vi "Teleop.vi"(10 "Match Info":T1={"Autonomous Elapsed Seconds"=0.0, "TeleOp Elapsed Seconds"=0.0, "Disabled Elapsed Seconds"=0.0, "Visited Autonomous"=FALSE, "Visited TeleOp"=FALSE, "Visited Disabled"=FALSE, "Autonomous Settings"={"Autonomous Style"=enum."Independent", "VI Refnum"=refnum}}, 11 "Call Context":T2) -> ()   [LabVIEW 2014]
doc: "This VI is called for each TeleOp packet received from the DS where the robot is not disabled. It is often used to read from the joysticks and update I/O or to update setpoints for timed control loops. It should complete and return within 20 milliseconds or it may miss DS packets."
uses:
  <vilib>/Rock Robotics/WPI/DriverStation/WPI_DriverStationDerivedRobotMode.ctl
  <vilib>/Rock Robotics/WPI/DriverStation/WPI_DriverStationMatch Info.ctl
  <vilib>/Rock Robotics/WPI/Solenoid/WPI_SolenoidValue.ctl
  <vilib>/Rock Robotics/WPI/Joystick/WPI_JoystickGetSetRefNum.vi
  Robot Global Data.vi
  Gyro/Gyro Global.vi
  <vilib>/Rock Robotics/WPI/Solenoid/WPI_SolenoidSetEnum.vi
  navX-MXP Library/navX-MXP IMU.lvlib
panel:
  out "error out":errorcluster
  out "up":bool
  out "same":bool
  out "manual?":bool
  out "t?":bool
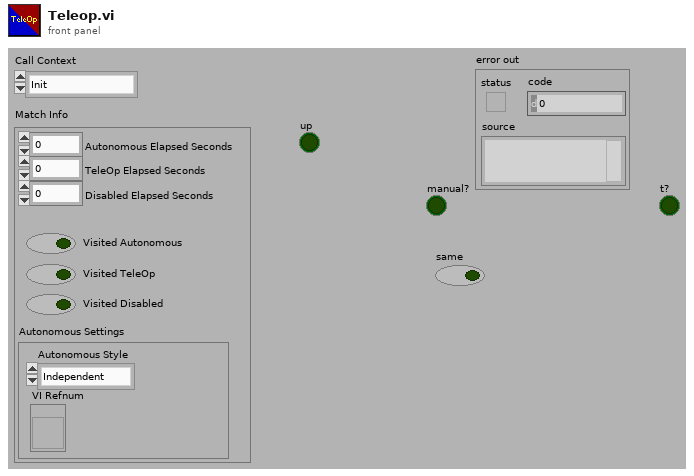
[diagram p1: front panel]
types:
  T1 = typedef "WPI_DriverStationMatch Info.ctl" = cluster{"Autonomous Elapsed Seconds":dbl, "TeleOp Elapsed Seconds":dbl, "Disabled Elapsed Seconds":dbl, "Visited Autonomous":bool, "Visited TeleOp":bool, "Visited Disabled":bool, "Autonomous Settings":cluster{"Autonomous Style":enum16{"Iterative", "Independent"}, "VI Refnum":refnum<vi>}}
  T2 = typedef "WPI_DriverStationDerivedRobotMode.ctl" = enum16{"Init", "Execute", "Stop"}
  T3 = typedef "WPI_SolenoidValue.ctl" = enum16{"Off", "On", "Forward", "Reverse"}
  T4 = typedef "WPI_JoystickDevRef.ctl" = cluster{"Device":T5}
  T5 = typedef "WPI_JoystickDeviceEnum.ctl" = enum16{"USB 0", "USB 1", "USB 2", "USB 3", "USB 4", "USB 5"}
  T6 = typedef "WPI_MotorControlDeviceRef.ctl" = cluster{"DeviceStatus":errorcluster, "Type":T7, "PWM":cluster{"Controller":T8, "PWM Channel":T9, "DeadBand":T10}, "CAN":cluster{"Device Number":u8, "Control Mode":T11, "Semaphore":T12, "Max Vout":dbl, "TalonSRX Control Mode":T13}, "Invert":bool, "TransformRef":T14, "InvTransformRef":T14}
  T7 = typedef "WPI_MotorControlType.ctl" = enum16{"PWM", "CAN", "CANTalonSRX"}
  T8 = typedef "FPGA_TypedefDigitalModule.ctl" = enum16{"Controller 1"}
  T9 = typedef "FPGA_DIOPWMChannel.ctl" = enum8{"PWM 0", "PWM 1", "PWM 2", "PWM 3", "PWM 4", "PWM 5", "PWM 6", "PWM 7", "PWM 8", "PWM 9", "PWM MXP 0", "PWM MXP 1", "PWM MXP 2", "PWM MXP 3", "PWM MXP 4", "PWM MXP 5", "PWM MXP 6", "PWM MXP 7", "PWM MXP 8", "PWM MXP 9", "Invalid"}
  T10 = typedef "WPI_PWMDeadband.ctl" = cluster{"Name":string, "maxPositivePwm":i32, "minPositivePwm":i32, "centerPwm":i32, "maxNegativePwm":i32, "minNegativePwm":i32, "angularRange":u16}
  T11 = typedef "WPI_CANJaguar_ControlMode.ctl" = enum8{"Percent VBus", "Current", "Speed", "Position", "Voltage"}
  T12 = typedef "Semaphore RefNum" = refnum<k1>
  T13 = typedef "WPI_CANTalonSRX_APIControlMode.ctl" = enum8{"Percent VBus", "Speed", "Position", "Slave", "Unchanged / Invalid"}
  T14 = typedef "WPI_PWMTransform_ConPane.ctl" = refnum<vi>
  T15 = typedef "navX-MXP IMU.lvlib/navX SPI DevRef.ctl" = cluster{"SPIDevRef":T16, "Board Information":T18, "Status":T19, "Offsets":cluster{"Yaw":dbl, "Quat W":dbl, "Quat X":dbl, "Quat Y":dbl, "Quat Z":dbl}, "Update Rate (4Hz-60Hz)":u8, "refnum name":string, "error":errorcluster}
  T16 = typedef "WPI_SPIDevRef.ctl" = cluster{"DevStatus":errorcluster, "Handle":i32, "Controller":T8, "SPI Bus":T17}
  T17 = typedef "spi_bus.ctl" = enum16{"SPI On-Board, CS0", "SPI On-Board, CS1", "SPI On-Board, CS2", "SPI On-Board, CS3", "SPI MXP", "Invalid"}
  T18 = typedef "navX-MXP IMU.lvlib/navX Board Information.ctl" = cluster{"WhoAmI (50 | 0x32)":u8, "Board Revision":u8, "Firmware Major Version":u8, "Firmware Minor Version":u8}
  T19 = typedef "navX-MXP IMU.lvlib/navX Status Data.ctl" = cluster{"Update Rate Hz":u8, "Accelerometer Full-Scale Range":u8, "Gyro Full-Scale Range":u16, "NAVX_OP_STATUS":T20, "NAVX_CAL_STATUS":T21, "NAVX_SELFTEST_STATUS":u8, "NAVX_SENSOR_STATUS":T22}
  T20 = typedef "navX-MXP IMU.lvlib/navX NAVX_OP_STATUS.ctl" = u8
  T21 = typedef "navX-MXP IMU.lvlib/navX NAVX_CAL_STATUS.ctl" = u8
  T22 = typedef "navX-MXP IMU.lvlib/navX NAVX_SENSOR_STATUS.ctl" = cluster{"MOVING":bool, "YAW_STABLE":bool, "MAG_DISTURBANCE":bool, "ALTITUDE_VALID":bool, "SEALEVEL_PRESS_SET":bool, "FUSED_HEADING_VALID":bool}
  T23 = typedef "navX-MXP IMU.lvlib/navX YPRH Data.ctl" = cluster{"Yaw":dbl, "Pitch":dbl, "Roll":dbl, "Heading":dbl}
  T24 = typedef "WPI_EncoderDevRef.ctl" = cluster{"DevStatus":errorcluster, "EncoderIndex":T25, "CounterIndex":T26, "DistancePerCount":dbl, "Decoding Type":T27}
  T25 = typedef "FPGA_EncoderIdx.ctl" = enum8{"Enc 0", "Enc 1", "Enc 2", "Enc 3", "Enc 4", "Enc 5", "Enc 6", "Enc 7", "Invalid"}
  T26 = typedef "FPGA_CounterCtrSystemIndex.ctl" = enum8{"Ctr 0", "Ctr 1", "Ctr 2", "Ctr 3", "Ctr 4", "Ctr 5", "Ctr 6", "Ctr 7", "Invalid"}
  T27 = typedef "WPI_EncoderType.ctl" = enum16{"1x", "2x", "4x"}
  T28 = typedef "WPI_SolenoidDevRef.ctl" = cluster{"DevStatus":errorcluster, "Pneumatics Control Module":u8, "Forward Solenoid Channel":T29, "Reverse Solenoid Channel":T29}
  T29 = typedef "WPI_SolenoidChannel.ctl" = enum8{"Solenoid 0", "Solenoid 1", "Solenoid 2", "Solenoid 3", "Solenoid 4", "Solenoid 5", "Solenoid 6", "Solenoid 7", "Invalid"}
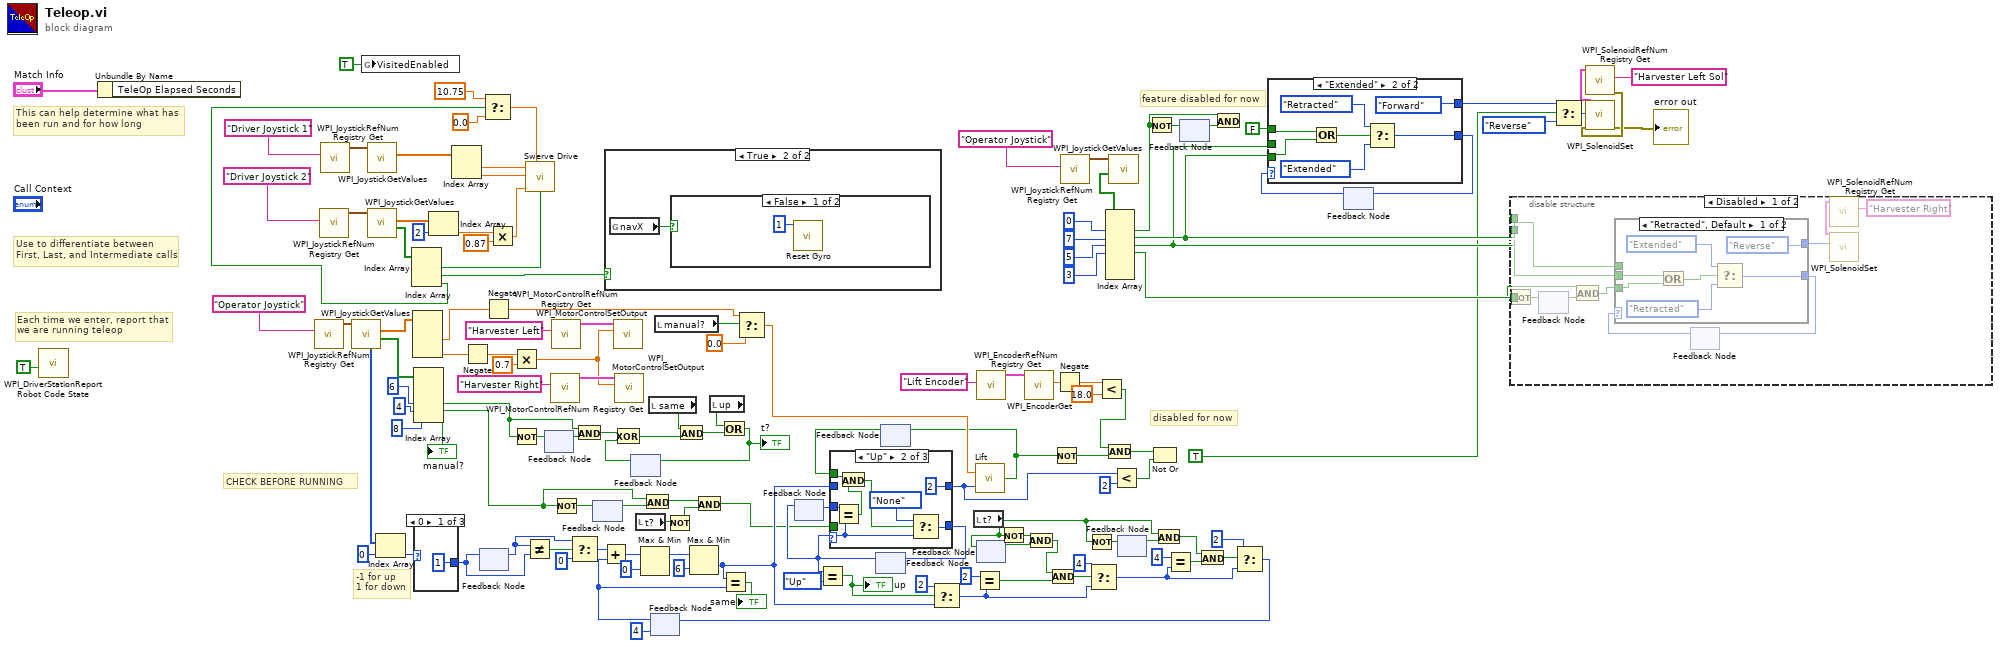
[diagram p0: block diagram]
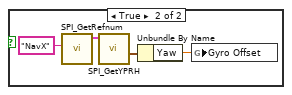
[diagram p3: hidden frame]
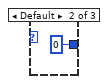
[diagram p4: hidden frame]
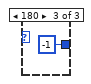
[diagram p5: hidden frame]
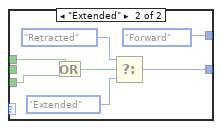
[diagram p6: hidden frame]
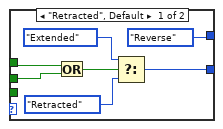
[diagram p8: hidden frame]
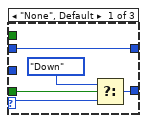
[diagram p9: hidden frame]
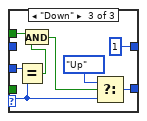
[diagram p10: hidden frame]
diagram:
  # "disabled for now"
  # "feature disabled for now"
  # "CHECK BEFORE RUNNING"
  # "-1 for up\n1 for down"
  # "Each time we enter, report that\nwe are running teleop"
  # "Use to differentiate between\nFirst, Last, and Intermediate calls"
  # "This can help determine what has\nbeen run and for how long"
  n1 = call <vilib>:"WPI_DriverStationReport Robot Code State.vi"("TeleOp"=TRUE ("Autonomous")) -> ()  [unwired: 10 in, 1 out]
  n2 = Unbundle By Name("Match Info") -> ()  [unwired: 1 out]
  n3 = call <vilib>:"WPI_JoystickRefNum Registry Get.vi"("refnum name"="Operator Joystick") -> ("JoystickDevRef"=w125:T4)  [unwired: 1 in, 9 out]
  n4 = call <vilib>:"WPI_JoystickRefNum Registry Get.vi"("refnum name"="Driver Joystick 2") -> ("JoystickDevRef"=w133:T4)  [unwired: 1 in, 9 out]
  n5 = call <vilib>:"WPI_JoystickRefNum Registry Get.vi"("refnum name"="Driver Joystick 1") -> ("JoystickDevRef"=w135:T4)  [unwired: 1 in, 9 out]
  n6 = call <vilib>:"WPI_JoystickGetValues.vi"("JoystickDevRef"=w125) -> ("Buttons"=w112:bool[], "Axes"=w124:dbl[], "POVs"=w119:i16[])  [unwired: 6 in, 2 out]
  n7 = global write "Gyro Global.vi" "VisitedEnabled"(TRUE ("VisitedEnabled")) -> ()
  n8 = call <vilib>:"WPI_JoystickGetValues.vi"("JoystickDevRef"=w135) -> ("Axes"=w131:dbl[])  [unwired: 6 in, 4 out]
  n9 = call <vilib>:"WPI_JoystickGetValues.vi"("JoystickDevRef"=w133) -> ("Buttons"=w127:bool[], "Axes"=w129:dbl[])  [unwired: 6 in, 3 out]
  n10 = Index Array(array=w119, index=0) -> (element=w44:i16)
  n11 = Index Array(array=w127) -> (element #1=w22:bool, element #2=w19:bool, element #3=w6:bool)  [unwired: 3 in]
  n12 = Index Array(array=w124) -> (element #2=w108:dbl, element #4=w109:dbl)  [unwired: 4 in, 2 out]
  n13 = Index Array(array=w112, index #3=6 ("index"), index #4=4 ("index"), index #5=8 ("index")) -> (element #3=w48:bool, element #4=w103:bool, element #5=→"manual?":bool)  [unwired: 2 in, 2 out]
  n14 = case shown="0" w44 {
    tunnel: [1 0 -1] -> w43
    frame 0 {
    }
    frame Default {
    }
    frame 180 {
    }
  }
  n15 = Index Array(array=w129, index=2) -> (element=w3:dbl)
  n16 = Index Array(array=w131) -> (element #1=w120:dbl, element #2=w130:dbl)  [unwired: 2 in]
  n17 = Negate(x=w109) -> (-x=w78:dbl)
  n18 = feedback-in #1(w43) -> ()
  n19 = feedback #1() -> (w45:i32)  [unwired: 1 in]
  n20 = Select(t=10.75 ("Rot. Point Y"), s=w6, f=0.0) -> (s? t:f=w4:dbl)
  n21 = Negate(x=w108) -> (-x=w73:dbl)
  n22 = Multiply(x=w3, y=0.87) -> (x*y=w2:dbl)
  n23 = Multiply(x=w78, y=0.7) -> (x*y=w21:dbl)
  n24 = Not(x=w48) -> (.not. x?=w82:bool)
  n25 = Not Equal?(x=w45, y=w43) -> (x != y?=w117:bool)
  n26 = call "Swerve Drive.vi"("X"=w120, "Rot. Point Y"=w4, "Y"=w130, "Z"=w2, "Robot-Centric"=w22) -> ()  [unwired: 11 in]
  n27 = feedback #2() -> (w83:bool)  [unwired: 1 in]
  n28 = feedback-in #2(w82) -> ()
  n29 = call <vilib>:"WPI_MotorControlRefNum Registry Get.vi"("refnum name"="Harvester Right") -> ("MotorControlDevRef"=w121:T6)  [unwired: 9 in, 1 out]
  n30 = call <vilib>:"WPI_MotorControlRefNum Registry Get.vi"("refnum name"="Harvester Left") -> ("MotorControlDevRef"=w122:T6)  [unwired: 9 in, 1 out]
  n31 = Not(x=w103) -> (.not. x?=w105:bool)
  n32 = Select(t=w45, s=w117, f=i16 0) -> (s? t:f=w52:i32)
  n33 = And(x=w48, y=w83) -> (x .and. y?=w81:bool)
  n34 = feedback #3() -> (w104:bool)  [unwired: 1 in]
  n35 = feedback-in #3(w105) -> ()
  n36 = case shown="True" w19 {
    frame False {
    }
    frame True {
      n37 = global read "Robot Global Data.vi" "navX"() -> (w141:bool)
      n38 = case shown="False" w141 {
        frame False {
          n39 = call "Reset Gyro.vi"("Gyro ID (1 or 2)"=1) -> ()  [unwired: 11 in]
        }
        frame True {
          n40 = call "SPI_GetRefnum.vi"("refnum name"="NavX") -> ("navX DevRef"=w144:T15)  [unwired: 9 in, 1 out]
          n41 = call "SPI_GetYPRH.vi"("navX DevRef"=w144) -> ("YPRH"=w143:T23)  [unwired: 8 in, 2 out]
          n42 = Unbundle By Name(w143) -> ("Yaw"=w146:dbl)
          n43 = global write "Robot Global Data.vi" "Gyro Offset"(w146) -> ()
        }
      }
    }
  }
  n44 = call <vilib>:"WPI_MotorControlSetOutput.vi"("Output"=w21, "MotorControlDevRef"=w122) -> ()  [unwired: 7 in, 3 out]
  n45 = call <vilib>:"WPI_MotorControlSetOutput.vi"("Output"=w21, "MotorControlDevRef"=w121) -> ()  [unwired: 7 in, 3 out]
  n46 = feedback #4() -> (w80:bool)  [unwired: 1 in]
  n47 = Exclusive Or(1:w80, 2:w81) -> (0:w36:bool)
  n48 = local read "t?"() -> (w28:bool)
  n49 = And(x=w103, y=w104) -> (x .and. y?=w30:bool)
  n50 = local read "same"() -> (w47:bool)
  n51 = feedback #5(i16 4 ("t")) -> (w51:i32)
  n52 = Add(x=w52, y=w51) -> (x+y=w84:i32)
  n53 = Max & Min(x=w84, y=i16 0) -> (max(x,y)=w110:i32)  [unwired: 1 out]
  n54 = local read "manual?"() -> (w74:bool)
  n55 = Not(x=w28) -> (.not. x?=w27:bool)
  n56 = And(x=w47, y=w36) -> (x .and. y?=w39:bool)
  n57 = Max & Min(x=w110, y=i16 6) -> (min(x,y)=w50:i32)  [unwired: 1 out]
  n58 = And(x=w30, y=w27) -> (x .and. y?=w29:bool)
  n59 = local read "up"() -> (w37:bool)
  n60 = Or(x=w37, y=w39) -> (x .or. y?=w38:bool)
  "t?" <- w38
  n61 = feedback-in #4(w38) -> ()
  n62 = Equal?(x=w50, y=w51) -> (x = y?=→"same":bool)
  n63 = Select(t=w73, s=w74, f=0.0) -> (s? t:f=w72:dbl)
  n64 = feedback #6() -> (w40:enum16{"None", "Up", "Down"})  [unwired: 1 in]
  n65 = feedback #7() -> (w41:enum16{"None", "Up", "Down"})  [unwired: 1 in]
  n66 = feedback-in #6(w41) -> ()
  n67 = Equal?(x=w41, y=enum16{"None", "Up", "Down"}."Up") -> (x = y?=w106:bool)
  "up" <- w106
  n68 = feedback #8() -> (w42:bool)  [unwired: 1 in]
  n69 = case shown="\"Up\"" w41 {
    selector: w41 -> [w149 w153 w162]
    tunnel: [w151 w159 w167] -> w86
    tunnel: [w148 i16 2 ("y") i16 1 ("y")] -> w23
    tunnel: w42 -> [_ w152 w164]
    tunnel: w50 -> [w148 _ _]
    tunnel: w29 -> [w147 _ _]
    tunnel: w40 -> [_ w154 w163]
    frame "None", Default {
      n70 = Select(t=enum16{"None", "Up", "Down"}."Down" ("f"), s=w147, f=w149) -> (s? t:f=w151:enum16{"None", "Up", "Down"})
    }
    frame "Up" {
      n71 = Equal?(x=w154, y=w153) -> (x = y?=w156:bool)
      n72 = And(x=w152, y=w156) -> (x .and. y?=w155:bool)
      n73 = Select(t=enum16{"None", "Up", "Down"}."None" ("f"), s=w155, f=w153) -> (s? t:f=w159:enum16{"None", "Up", "Down"})
    }
    frame "Down" {
      n74 = Equal?(x=w163, y=w162) -> (x = y?=w161:bool)
      n75 = And(x=w164, y=w161) -> (x .and. y?=w160:bool)
      n76 = Select(t=enum16{"None", "Up", "Down"}."Up" ("f"), s=w160, f=w162) -> (s? t:f=w167:enum16{"None", "Up", "Down"})
    }
  }
  n77 = feedback-in #7(w86) -> ()
  n78 = Select(t=i16 2, s=w106, f=w50) -> (s? t:f=w66:i32)
  n79 = local read "t?"() -> (w60:bool)
  n80 = Equal?(x=i16 2, y=w66) -> (x = y?=w68:bool)
  n81 = call "Lift.vi"("Level"=w23, "Manual"=w72) -> ("At Level"=w34:bool)
  n82 = feedback-in #8(w34) -> ()
  n83 = call <vilib>:"WPI_EncoderRefNum Registry Get.vi"("refnum name"="Lift Encoder") -> ("EncoderDevRef"=w14:T24)  [unwired: 9 in, 1 out]
  n84 = feedback #9() -> (w64:bool)  [unwired: 1 in]
  n85 = feedback-in #9(w60) -> ()
  n86 = Not(x=w60) -> (.not. x?=w65:bool)
  n87 = call <vilib>:"WPI_EncoderGet.vi"("EncoderDevRef"=w14) -> ("Distance"=w12:dbl)  [unwired: 5 in, 5 out]
  n88 = And(x=w65, y=w64) -> (x .and. y?=w63:bool)
  n89 = And(x=w63, y=w68) -> (x .and. y?=w67:bool)
  n90 = Not(x=w34) -> (.not. x?=w13:bool)
  n91 = Negate(x=w12) -> (-x=w11:dbl)
  n92 = call <vilib>:"WPI_JoystickRefNum Registry Get.vi"("refnum name"="Operator Joystick") -> ("JoystickDevRef"=w97:T4)  [unwired: 1 in, 9 out]
  n93 = Not(x=w60) -> (.not. x?=w62:bool)
  n94 = Select(t=i16 4 ("y"), s=w67, f=w66) -> (s? t:f=w55:i32)
  n95 = Less?(x=w11, y=18.0) -> (x < y?=w9:bool)
  n96 = And(x=w9, y=w13) -> (x .and. y?=w26:bool)
  n97 = call <vilib>:"WPI_JoystickGetValues.vi"("JoystickDevRef"=w97) -> ("Buttons"=w95:bool[])  [unwired: 6 in, 4 out]
  n98 = Index Array(array=w95, index #1=0 ("index"), index #2=7 ("index"), index #3=5 ("index"), index #4=3 ("index")) -> (element #1=w94:bool, element #2=w93:bool, element #3=w92:bool, element #4=w87:bool)  [unwired: 3 in, 3 out]
  n99 = Less?(x=w23, y=2) -> (x < y?=w24:bool)
  n100 = feedback #10() -> (w61:bool)  [unwired: 1 in]
  n101 = feedback-in #10(w62) -> ()
  n102 = Not(x=w94) -> (.not. x?=w100:bool)
  n103 = Not Or(1:w24, 2:w26) -> ()  [unwired: 1 out]
  n104 = And(x=w60, y=w61) -> (x .and. y?=w57:bool)
  n105 = Equal?(x=i16 4, y=w55) -> (x = y?=w58:bool)
  n106 = feedback #11() -> (w99:bool)  [unwired: 1 in]
  n107 = feedback-in #11(w100) -> ()
  n108 = And(x=w57, y=w58) -> (x .and. y?=w56:bool)
  n109 = And(x=w94, y=w99) -> ()  [unwired: 1 out]
  n110 = Select(t=i16 2, s=w56, f=w55) -> (s? t:f=w53:i32)
  n111 = feedback-in #5(w53) -> ()
  n112 = feedback #12() -> (w101:enum16{"Retracted", "Extended"})  [unwired: 1 in]
  n113 = case shown="\"Extended\"" w101 {
    tunnel: [WPI_SolenoidValue."Reverse" ("Solenoid Left") WPI_SolenoidValue."Forward" ("Solenoid Left")] -> w33
    tunnel: [w171 w177] -> w35
    tunnel: FALSE -> [w169 w178]
    tunnel: w93 -> [_ w175]
    tunnel: w92 -> [w168 _]
    frame "Retracted", Default {
      n114 = Or(x=w169, y=w168) -> (x .or. y?=w174:bool)
      n115 = Select(t=enum16{"Retracted", "Extended"}."Extended", s=w174, f=enum16{"Retracted", "Extended"}."Retracted") -> (s? t:f=w171:enum16{"Retracted", "Extended"})
    }
    frame "Extended" {
      n116 = Or(x=w178, y=w175) -> (x .or. y?=w181:bool)
      n117 = Select(t=enum16{"Retracted", "Extended"}."Retracted", s=w181, f=enum16{"Retracted", "Extended"}."Extended") -> (s? t:f=w177:enum16{"Retracted", "Extended"})
    }
  }
  n118 = feedback-in #12(w35) -> ()
  n119 = disable-structure shown="Disabled" {
    disable-tunnel: w93 -> [w184 _]
    disable-tunnel: w92 -> [w183 _]
    disable-tunnel: w87 -> [w182 _]
    frame Disabled {
      n120 = Not(x=w182) -> (.not. x?=w189:bool)
      n121 = feedback #13() -> (w190:bool)  [unwired: 1 in]
      n122 = feedback-in #13(w189) -> ()
      n123 = And(x=w182, y=w190) -> (x .and. y?=w191:bool)
      n124 = feedback #14() -> (w188:enum16{"Retracted", "Extended"})  [unwired: 1 in]
      n125 = case shown="\"Retracted\", Default" w188 {
        tunnel: [WPI_SolenoidValue."Reverse" ("Solenoid Left") WPI_SolenoidValue."Forward" ("Solenoid Left")] -> w186
        tunnel: [w196 w203] -> w187
        tunnel: w191 -> [w194 w201]
        tunnel: w184 -> [_ w200]
        tunnel: w183 -> [w193 _]
        frame "Retracted", Default {
          n126 = Or(x=w193, y=w194) -> (x .or. y?=w199:bool)
          n127 = Select(t=enum16{"Retracted", "Extended"}."Extended", s=w199, f=enum16{"Retracted", "Extended"}."Retracted") -> (s? t:f=w196:enum16{"Retracted", "Extended"})
        }
        frame "Extended" {
          n128 = Or(x=w200, y=w201) -> (x .or. y?=w206:bool)
          n129 = Select(t=enum16{"Retracted", "Extended"}."Retracted", s=w206, f=enum16{"Retracted", "Extended"}."Extended") -> (s? t:f=w203:enum16{"Retracted", "Extended"})
        }
      }
      n130 = feedback-in #14(w187) -> ()
      n131 = call <vilib>:"WPI_SolenoidRefNum Registry Get.vi"("refnum name"="Harvester Right") -> ("SolenoidDevRef"=w192:T28)  [unwired: 9 in, 1 out]
      n132 = call-poly <vilib>:"WPI_SolenoidSet.vi"("Value"=w186, "SolenoidDevRef"=w192) -> ()  [unwired: 8 in, 2 out]
    }
    frame Enabled {
    }
  }
  n133 = Select(t=w33, s=TRUE, f=WPI_SolenoidValue."Reverse") -> (s? t:f=w32:T3)
  n134 = call <vilib>:"WPI_SolenoidRefNum Registry Get.vi"("refnum name"="Harvester Left Sol") -> ("error out"=w17:errorcluster, "SolenoidDevRef"=w98:T28)  [unwired: 9 in]
  n135 = call-poly <vilib>:"WPI_SolenoidSet.vi"("error in (no error)"=w17, "Value"=w32, "SolenoidDevRef"=w98) -> ("error out"=→"error out":errorcluster)  [unwired: 7 in, 1 out]
